vi "LinSpace (start-stop-step).vi"(3 "Step":dbl, 4 "Stop":dbl, 5 "Start":dbl) -> (0 "error out":errorcluster, 1 "Array":dbl[](array[numeric]))   [LabVIEW 2020]
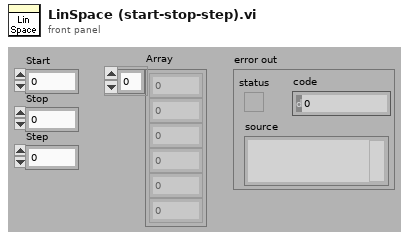
[diagram p1: front panel]
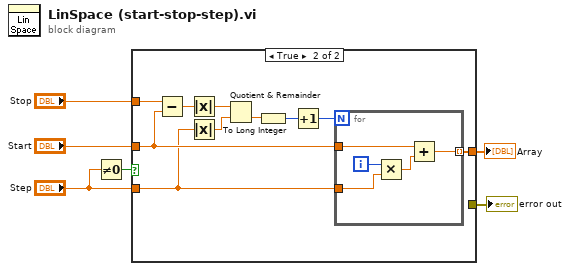
[diagram p0: block diagram]
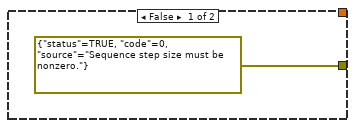
[diagram p2: hidden frame]
diagram:
  n1 = Not Equal To 0?(x="Step") -> (x != 0?=w2:bool)
  n2 = case shown="True" w2 {
    tunnel: "Start" -> [_ w15]
    tunnel: [_ w17] -> w5
    tunnel: "Stop" -> [_ w16]
    tunnel: "Step" -> [_ w12]
    tunnel: [errorcluster {"status"=TRUE, "code"=0, "source"="Sequence step size must be nonzero."} ("error out") _] -> w1
    frame False {
    }
    frame True {
      n3 = Subtract(x=w16, y=w15) -> (x-y=w14:dbl)
      n4 = Absolute Value(x=w14) -> (abs(x)=w13:dbl)
      n5 = Absolute Value(x=w12) -> (abs(x)=w11:dbl)
      n6 = Quotient & Remainder(x=w13, y=w11) -> (floor(x/y)=w10:dbl)  [unwired: 1 out]
      n7 = To Long Integer(number=w10) -> (32bit integer=w9:i32)
      n8 = Increment(x=w9) -> (x+1=w8:i32)
      n9 = for {
        N: w8 -> [_]
        tunnel: w15 -> [w21]
        tunnel: w12 -> [w19]
        tunnel: [w18] -> w17 mode=indexing
        i -> [w22]
        n10 = Multiply(x=w22, y=w19) -> (x*y=w20:dbl)
        n11 = Add(x=w21, y=w20) -> (x+y=w18:dbl)
      }
    }
  }
  "Array" <- w5
  "error out" <- w1
